vi "Write Display_Ref.vi"(8 "error in (no error)":errorcluster, 10 "Display_Ref":refnum<vi>, 11 "SwitchMatrix in":refnum<class "SwitchMatrix.lvclass">) -> (0 "error out":errorcluster, 3 "SwitchMatrix out":refnum<class "SwitchMatrix.lvclass">)   [LabVIEW 2019, in "SwitchMatrix.lvlib" / "SwitchMatrix.lvclass"]
uses:
  Library/SwitchMatrix.lvclass
  Library/SwitchMatrix.lvclass/SwitchMatrix.ctl
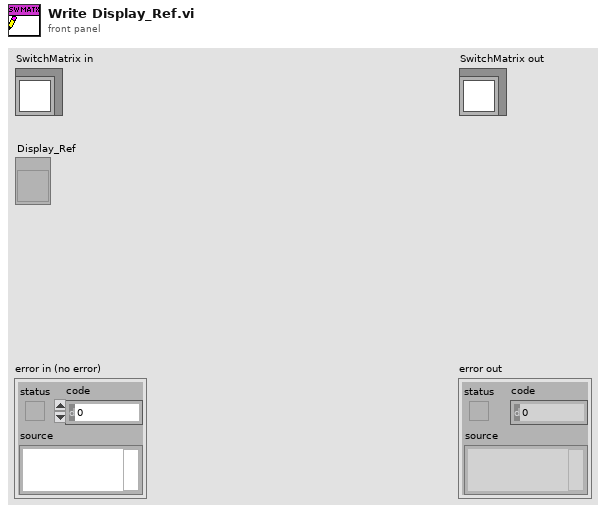
[diagram p1: front panel]
types:
  T1 = typedef "SwitchMatrix.lvlib/SwitchMatrix.lvclass/Topology_Mode.ctl" = enum16{"Single", "Dual", "Quad", "Octal", "Sixteen"}
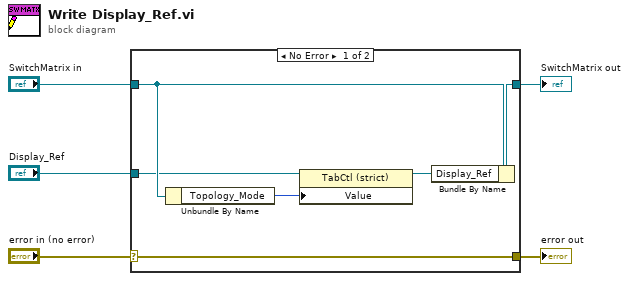
[diagram p0: block diagram]
diagram:
  n1 = case shown="No Error" "error in (no error)" {
    selector: "error in (no error)" -> [w11 w12]
    tunnel: [w11 w12] -> w4
    tunnel: [w10 w13] -> w2
    tunnel: "SwitchMatrix in" -> [w9 w13]
    tunnel: "Display_Ref" -> [w8 _]
    frame No Error {
      n2 = Unbundle By Name(w9) -> ("Topology_Mode"=w6:T1)
      n3 = property class="TabCtl (strict)"(reference=w8, "Value"=w6) -> (reference out=w7:refnum<vi>)  [unwired: 1 in, 1 out]
      n4 = Bundle By Name(cluster=w9, "Display_Ref"=w7) -> (w10:refnum<class "SwitchMatrix.lvclass">)
    }
    frame Error {
    }
  }
  "error out" <- w4
  "SwitchMatrix out" <- w2
